vi "Startup.vi"() -> (3 "Good":bool)   [LabVIEW 2011]
uses:
  <vilib>/Rock Robotics/SystemInterfaces/WatchDog/FPGA_WatchdogDevRef.ctl
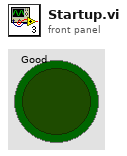
[diagram p1: front panel]
types:
  T1 = typedef "WPI_EncoderDevRef.ctl" = cluster{"DevStatus":errorcluster, "EncoderIndex":T2, "CounterIndex":T3, "DistancePerCount":dbl, "Decoding Type":T4}
  T2 = typedef "FPGA_EncoderIdx.ctl" = enum8{"Enc 0", "Enc 1", "Enc 2", "Enc 3", "Invalid"}
  T3 = typedef "FPGA_CounterCtrSystemIndex.ctl" = enum8{"Ctr 0", "Ctr 1", "Ctr 2", "Ctr 3", "Ctr 4", "Ctr 5", "Ctr 6", "Ctr 7", "Invalid"}
  T4 = typedef "WPI_EncoderType.ctl" = enum16{"1x", "2x", "4x"}
  T5 = typedef "FPGA_WatchdogDevRef.ctl" = cluster{"DevStatus":errorcluster}
  T6 = typedef "WPI_MotorControlDeviceRef.ctl" = cluster{"DeviceStatus":errorcluster, "Type":enum16{"PWM", "CAN"}, "PWM":cluster{"Digital Module":T7, "PWM Channel":T8, "DeadBand":T9}, "CAN":cluster{"Device Number":u8, "Control Mode":T10, "Semaphore":T11, "Max Vout":dbl}, "Invert":bool, "TransformRef":T12, "InvTransformRef":T12}
  T7 = typedef "FPGA_TypedefDigitalModule.ctl" = enum16{"Digital Module 1", "Digital Module 2"}
  T8 = typedef "FPGA_DIOPWMChannel.ctl" = enum8{"PWM 1", "PWM 2", "PWM 3", "PWM 4", "PWM 5", "PWM 6", "PWM 7", "PWM 8", "PWM 9", "PWM 10", "Invalid"}
  T9 = typedef "WPI_PWMDeadband.ctl" = cluster{"Name":string, "maxPositivePwm":i32, "minPositivePwm":i32, "centerPwm":i32, "maxNegativePwm":i32, "minNegativePwm":i32, "angularRange":u16}
  T10 = typedef "WPI_CANJaguar_ControlMode.ctl" = enum8{"Percent VBus", "Current", "Speed", "Position", "Voltage"}
  T11 = typedef "Semaphore RefNum" = refnum<k1>
  T12 = typedef "WPI_PWMTransform_ConPane.ctl" = refnum<vi>
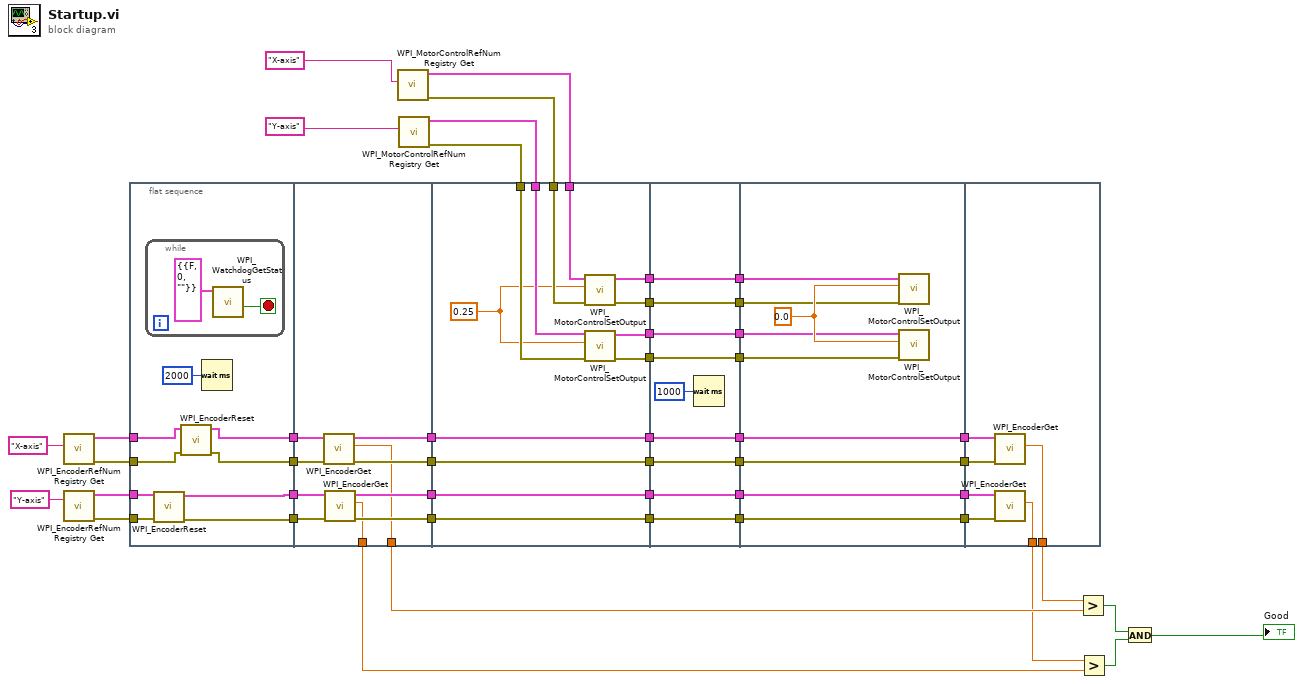
[diagram p0: block diagram]
diagram:
  n1 = call <vilib>:"WPI_EncoderRefNum Registry Get.vi"("refnum name"="X-axis") -> ("error out"=w11:errorcluster, "EncoderDevRef"=w12:T1)  [unwired: 9 in]
  n2 = call <vilib>:"WPI_EncoderRefNum Registry Get.vi"("refnum name"="Y-axis") -> ("error out"=w9:errorcluster, "EncoderDevRef"=w10:T1)  [unwired: 9 in]
  n3 = flat-sequence {
    tunnel: w9 -> [w51]
    tunnel: w10 -> [w50]
    tunnel: w11 -> [w54]
    tunnel: w12 -> [w55]
    tunnel: [w53] -> w42
    tunnel: [w52] -> w41
    tunnel: [w49] -> w40
    tunnel: [w48] -> w39
    tunnel: [w64] -> w38
    tunnel: [w63] -> w37
    tunnel: [w62] -> w36
    tunnel: [w61] -> w35
    tunnel: [w60] -> w8
    tunnel: [w59] -> w5
    tunnel: w42 -> [w68]
    tunnel: w41 -> [w67]
    tunnel: w40 -> [w66]
    tunnel: w39 -> [w65]
    tunnel: w47 -> [w81]
    tunnel: w46 -> [w80]
    tunnel: w45 -> [w79]
    tunnel: w44 -> [w78]
    tunnel: [w76] -> w34
    tunnel: w38 -> [w76]
    tunnel: [w75] -> w33
    tunnel: w37 -> [w75]
    tunnel: w36 -> [w74]
    tunnel: [w74] -> w32
    tunnel: w35 -> [w73]
    tunnel: [w73] -> w31
    tunnel: [w72] -> w30
    tunnel: [w71] -> w29
    tunnel: [w70] -> w28
    tunnel: [w69] -> w27
    tunnel: w34 -> [w90]
    tunnel: [w90] -> w26
    tunnel: w33 -> [w89]
    tunnel: [w89] -> w25
    tunnel: w32 -> [w88]
    tunnel: [w88] -> w24
    tunnel: w31 -> [w87]
    tunnel: [w87] -> w23
    tunnel: w30 -> [w85]
    tunnel: [w85] -> w22
    tunnel: w29 -> [w84]
    tunnel: [w84] -> w21
    tunnel: w28 -> [w83]
    tunnel: [w83] -> w20
    tunnel: [w82] -> w19
    tunnel: w27 -> [w82]
    tunnel: w26 -> [w99]
    tunnel: [w99] -> w18
    tunnel: w25 -> [w98]
    tunnel: [w98] -> w17
    tunnel: w24 -> [w97]
    tunnel: [w97] -> w16
    tunnel: w23 -> [w96]
    tunnel: [w96] -> w15
    tunnel: w22 -> [w94]
    tunnel: w21 -> [w93]
    tunnel: w20 -> [w92]
    tunnel: w19 -> [w91]
    tunnel: w18 -> [w105]
    tunnel: w17 -> [w104]
    tunnel: w16 -> [w103]
    tunnel: w15 -> [w102]
    tunnel: [w101] -> w7
    tunnel: [w100] -> w6
    frame #0 {
      n4 = while {
        stop <- w58 stop-if-true
        n5 = call <vilib>:"WPI_WatchdogGetStatus.vi"("WatchdogDevRef"=T5 {"DevStatus"={"status"=FALSE, "code"=0, "source"=""}}) -> ("SystemActive"=w58:bool)  [unwired: 7 in, 3 out]
      }
      n6 = call <vilib>:"WPI_EncoderReset.vi"("error in (no error)"=w51, "EncoderDevRef"=w50) -> ("error out"=w48:errorcluster, "EncoderDevRef"=w49:T1)  [unwired: 8 in]
      n7 = call <vilib>:"WPI_EncoderReset.vi"("error in (no error)"=w54, "EncoderDevRef"=w55) -> ("error out"=w52:errorcluster, "EncoderDevRef"=w53:T1)  [unwired: 8 in]
      n8 = Wait (ms)(milliseconds to wait=u32 2000) -> ()  [unwired: 1 out]
    }
    frame #1 {
      n9 = call <vilib>:"WPI_EncoderGet.vi"("error in (no error)"=w67, "EncoderDevRef"=w68) -> ("error out"=w63:errorcluster, "Distance"=w60:dbl, "EncoderDevRef"=w64:T1)  [unwired: 4 in, 3 out]
      n10 = call <vilib>:"WPI_EncoderGet.vi"("error in (no error)"=w65, "EncoderDevRef"=w66) -> ("error out"=w61:errorcluster, "Distance"=w59:dbl, "EncoderDevRef"=w62:T1)  [unwired: 4 in, 3 out]
    }
    frame #2 {
      w77 = 0.25 ("Output")
      n11 = call <vilib>:"WPI_MotorControlSetOutput.vi"("error in (no error)"=w80, "Output"=w77, "MotorControlDevRef"=w81) -> ("error out"=w69:errorcluster, "MotorControlDevRef"=w72:T6)  [unwired: 7 in]
      n12 = call <vilib>:"WPI_MotorControlSetOutput.vi"("error in (no error)"=w78, "Output"=w77, "MotorControlDevRef"=w79) -> ("error out"=w70:errorcluster, "MotorControlDevRef"=w71:T6)  [unwired: 7 in]
    }
    frame #3 {
      n13 = Wait (ms)(milliseconds to wait=u32 1000) -> ()  [unwired: 1 out]
    }
    frame #4 {
      w95 = 0.0 ("Output")
      n14 = call <vilib>:"WPI_MotorControlSetOutput.vi"("error in (no error)"=w91, "Output"=w95, "MotorControlDevRef"=w94) -> ()  [unwired: 7 in, 2 out]
      n15 = call <vilib>:"WPI_MotorControlSetOutput.vi"("error in (no error)"=w92, "Output"=w95, "MotorControlDevRef"=w93) -> ()  [unwired: 7 in, 2 out]
    }
    frame #5 {
      n16 = call <vilib>:"WPI_EncoderGet.vi"("error in (no error)"=w104, "EncoderDevRef"=w105) -> ("Distance"=w101:dbl)  [unwired: 4 in, 5 out]
      n17 = call <vilib>:"WPI_EncoderGet.vi"("error in (no error)"=w102, "EncoderDevRef"=w103) -> ("Distance"=w100:dbl)  [unwired: 4 in, 5 out]
    }
  }
  n18 = call <vilib>:"WPI_MotorControlRefNum Registry Get.vi"("refnum name"="X-axis") -> ("error out"=w46:errorcluster, "MotorControlDevRef"=w47:T6)  [unwired: 9 in]
  n19 = call <vilib>:"WPI_MotorControlRefNum Registry Get.vi"("refnum name"="Y-axis") -> ("error out"=w44:errorcluster, "MotorControlDevRef"=w45:T6)  [unwired: 9 in]
  n20 = Greater?(x=w7, y=w8) -> (0:w4:bool)
  n21 = Greater?(x=w6, y=w5) -> (0:w3:bool)
  n22 = And(x=w4, y=w3) -> (x .and. y?=→"Good":bool)
